vi "Measure Multi.vi"(7 "Config for Immediate Measure?(T)":bool=TRUE, 8 "error in (no error)":errorcluster, 9 "Max Time (-1ms)":i32=-1, 10 "Measurements to Acquire(1)":i32=1 min=0, 11 "NI DMM Driver in":refnum<class "DMM.NI.lvclass">) -> (0 "error dub":errorcluster, 2 "Measurements":dbl[](array[numeric]), 3 "NI DMM Driver out":refnum<class "DMM.NI.lvclass">)   [LabVIEW 2020, in "NI DMM Driver.lvlib" / "DMM.NI.lvclass"]
doc: "Perform multiple measurement on the DMM. \nTimeout should not result in errors.\nMeasurements should only contain actual completed measurements."
uses:
  DMM.NI.lvclass
  <instrlib>/niDMM/nidmm.llb/niDMM Sample Trigger.ctl
  Controls/Ctl_MultiReadConfig.ctl
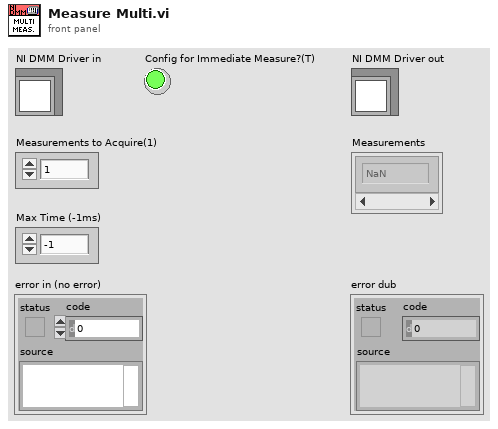
[diagram p1: front panel]
types:
  T1 = typedef "NI DMM Driver.lvlib/Ctl_MultiReadConfig.ctl" = cluster{"Trigger Count":i32, "Sample Count":i32, "Sample Trigger":T2, "Sample Interval (sec)":dbl}
  T2 = typedef "niDMM Sample Trigger.ctl" = enum16{"Immediate", "External", "TTL 0", "TTL 1", "TTL 2", "TTL 3", "TTL 4", "TTL 5", "TTL 6", "Interval", "Software", "TTL 7", "PXI Star", "LBR Trig 1", "Aux Trig 1"}
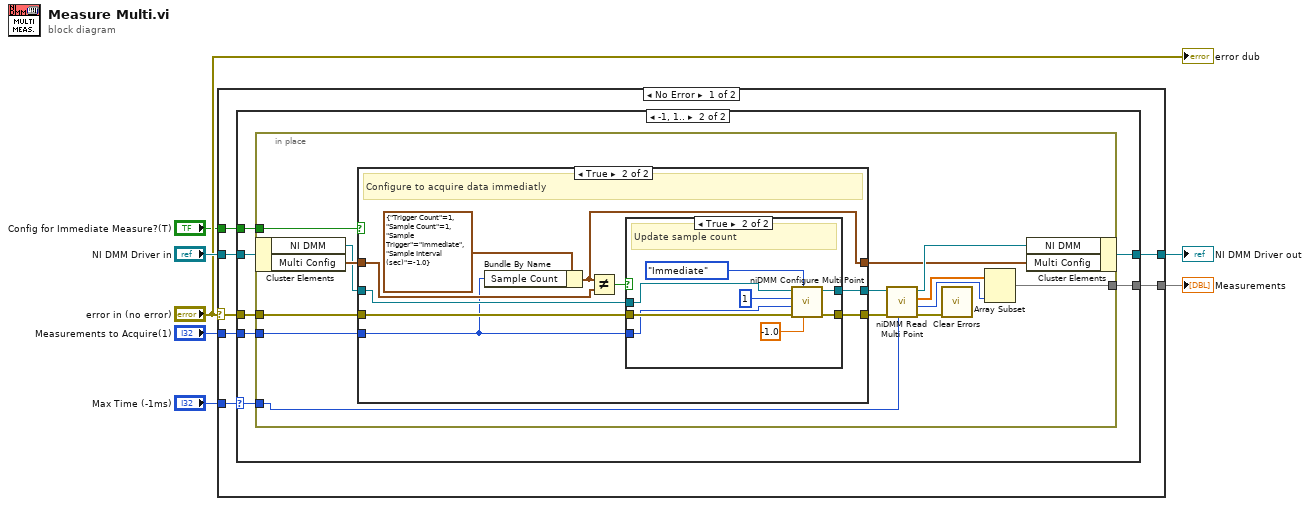
[diagram p0: block diagram]
diagram:
  n1 = case shown="No Error" "error in (no error)" {
    selector: "error in (no error)" -> [w12 _]
    tunnel: [w13 w59] -> w2
    tunnel: "NI DMM Driver in" -> [w14 w59]
    tunnel: "Measurements to Acquire(1)" -> [w11 _]
    tunnel: "Max Time (-1ms)" -> [w10 _]
    tunnel: [w9 _] -> w3
    tunnel: "Config for Immediate Measure?(T)" -> [w8 _]
    frame No Error {
      n2 = case shown="-1, 1.." w10 {
        selector: w10 -> [_ w18]
        tunnel: w14 -> [w15 w22]
        tunnel: [w15 w21] -> w13
        tunnel: w12 -> [_ w20]
        tunnel: w11 -> [_ w19]
        tunnel: [_ w17] -> w9
        tunnel: w8 -> [_ w16]
        frame 0, Default {
        }
        frame -1, 1.. {
          n3 = in-place {
            in-place-border: w20 -> [w26]
            in-place-border: w19 -> [w25]
            in-place-border: w18 -> [w35]
            in-place-border: [w33] -> w17
            in-place-border: w16 -> [w24]
            n4 = in-place-cluster #1(w22) -> ("NI DMM"=w28:refnum<k15>, "Multi Config"=w30:T1)
            n5 = case shown="True" w24 {
              tunnel: w30 -> [w39 w48]
              tunnel: [w37 w47] -> w29
              tunnel: w28 -> [w37 w46]
              tunnel: [w38 w45] -> w27
              tunnel: w26 -> [w38 w44]
              tunnel: w25 -> [_ w41]
              tunnel: [w39 w42] -> w23
              frame False {
                # "Do not change configuration"
              }
              frame True {
                # "Configure to acquire data immediatly"
                n6 = Bundle By Name(cluster=T1 {"Trigger Count"=1, "Sample Count"=1, "Sample Trigger"=enum."Immediate", "Sample Interval (sec)"=-1.0} ("Multi Measure"), "Sample Count"=w41) -> (w42:T1)
                n7 = Not Equal?(x=w42, y=w48) -> (x != y?=w40:bool)
                n8 = case shown="True" w40 {
                  tunnel: [w50 w52] -> w47
                  tunnel: w46 -> [w50 w55]
                  tunnel: [w49 w53] -> w45
                  tunnel: w44 -> [w49 w54]
                  tunnel: w41 -> [_ w51]
                  frame False {
                    # "Sample count is OK"
                  }
                  frame True {
                    # "Update sample count"
                    n9 = call <instrlib>:"niDMM Configure Multi Point.vi"("Sample Interval (sec)"=-1.0, "Sample Trigger"=niDMM_Sample_Trigger."Immediate", "error in (no error)"=w54, "Sample Count"=w51, "Trigger Count"=1, "instrument handle"=w55) -> ("error out"=w53:errorcluster, "instrument handle out"=w52:refnum<k15>)  [unwired: 4 in]
                  }
                }
              }
            }
            n10 = call <instrlib>:"niDMM Read Multi Point.vi"("Maximum Time (msec)"=w35, "error in (no error)"=w27, "instrument handle"=w29) -> ("error out"=w32:errorcluster, "Actual Number"=w31:i32, "Measurements"=w34:dbl[], "instrument handle out"=w36:refnum<k15>)  [unwired: 5 in]
            n11 = call <vilib>:"Clear Errors.vi"("error in (no error)"=w32) -> ()  [unwired: 5 in, 2 out]
            n12 = Array Subset(array=w34, length=w31) -> (w33:dbl[])  [unwired: 1 in]
            n13 = in-place-cluster #1("NI DMM"=w36, "Multi Config"=w23) -> (w21:refnum<class "DMM.NI.lvclass">)
          }
        }
      }
    }
    frame Error {
    }
  }
  "NI DMM Driver out" <- w2
  "Measurements" <- w3
  "error dub" <- "error in (no error)"
